vi "概率随机数生成.vi"(10 "数值比例":string, 11 "数值范围":string) -> (0 "浮点数（字符串）":string, 1 "整数（字符串）":string, 2 "浮点数":dbl, 3 "整数":i32)   [LabVIEW 2013]
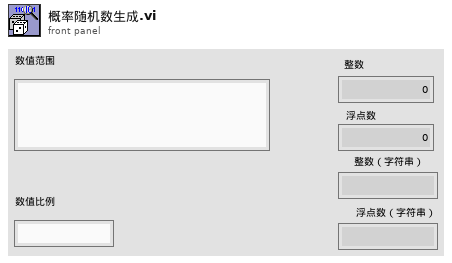
[diagram p1: front panel]
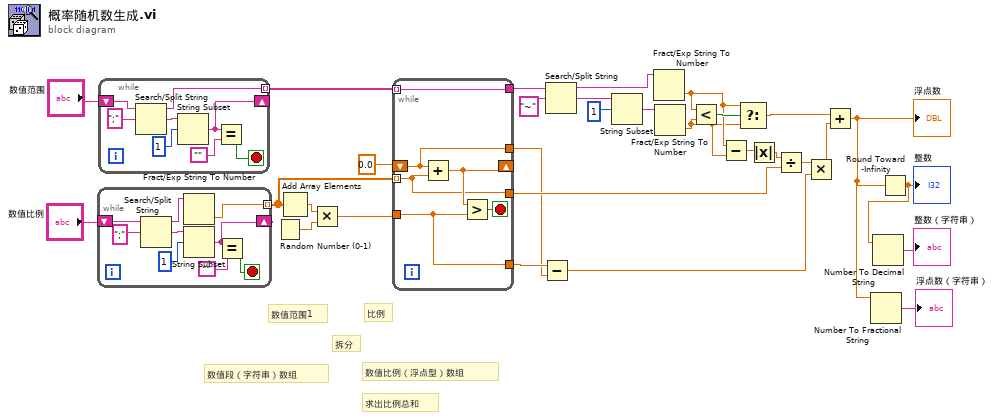
[diagram p0: block diagram]
diagram:
  # "求出比例总和"
  # "数值比例（浮点型）数组"
  # "数值段（字符串）数组"
  # "拆分"
  # "比例"
  # "数值范围1"
  n1 = while {
    tunnel: [w36] -> w26 mode=indexing
    shift-right: [w33] -> _
    shift-left: "数值比例" -> [w39]
    stop <- w31 stop-if-true
    n2 = Search/Split String(string=w39, search string/char (-)=";" ("搜索字符串/字符(-)")) -> (substring before match=w37:string, match + rest of string=w35:string)  [unwired: 1 in, 1 out]
    n3 = Fract/Exp String To Number(string=w37) -> (number=w36:dbl)  [unwired: 3 in, 1 out]
    n4 = String Subset(string=w35, offset (0)=1 ("偏移量(0)")) -> (substring=w33:string)  [unwired: 1 in]
    n5 = Equal?(x=w33, y="") -> (x = y?=w31:bool)
  }
  n6 = while {
    shift-right: [w43] -> _
    shift-left: "数值范围" -> [w47]
    tunnel: [w40] -> w23 mode=indexing
    stop <- w41 stop-if-true
    n7 = Search/Split String(string=w47, search string/char (-)=";" ("搜索字符串/字符(-)")) -> (substring before match=w40:string, match + rest of string=w45:string)  [unwired: 1 in, 1 out]
    n8 = String Subset(string=w45, offset (0)=1 ("偏移量(0)")) -> (substring=w43:string)  [unwired: 1 in]
    n9 = Equal?(x=w43, y="") -> (x = y?=w41:bool)
  }
  n10 = Random Number (0-1)() -> (number: 0 to 1=w27:dbl)
  n11 = Add Array Elements(numeric array=w26) -> (sum=w28:dbl)
  n12 = Multiply(x=w28, y=w27) -> (x*y=w24:dbl)
  n13 = while {
    tunnel: w24 -> [w50]
    tunnel: w26 -> [w49] mode=indexing
    shift-right: [w52] -> _
    shift-left: 0.0 -> [w48]
    tunnel: w23 -> [w51] mode=indexing
    tunnel: [w51] -> w22
    tunnel: [w50] -> w7
    tunnel: [w49] -> w10
    tunnel: [w48] -> w6
    stop <- w53 stop-if-true
    n14 = Add(x=w48, y=w49) -> (x+y=w52:dbl)
    n15 = Greater?(x=w52, y=w50) -> (0:w53:bool)
  }
  n16 = Subtract(x=w7, y=w6) -> (x-y=w5:dbl)
  n17 = Search/Split String(string=w22, search string/char (-)="~" ("搜索字符串/字符(-)")) -> (substring before match=w16:string, match + rest of string=w20:string)  [unwired: 1 in, 1 out]
  n18 = String Subset(string=w20, offset (0)=1 ("偏移量(0)")) -> (substring=w18:string)  [unwired: 1 in]
  n19 = Fract/Exp String To Number(string=w16) -> (number=w14:dbl)  [unwired: 3 in, 1 out]
  n20 = Fract/Exp String To Number(string=w18) -> (number=w13:dbl)  [unwired: 3 in, 1 out]
  n21 = Less?(x=w14, y=w13) -> (x < y?=w17:bool)
  n22 = Subtract(x=w14, y=w13) -> (x-y=w12:dbl)
  n23 = Select(t=w14, s=w17, f=w13) -> (s? t:f=w15:dbl)
  n24 = Absolute Value(x=w12) -> (abs(x)=w11:dbl)
  n25 = Divide(x=w11, y=w10) -> (x/y=w9:dbl)
  n26 = Multiply(x=w9, y=w5) -> (x*y=w8:dbl)
  n27 = Add(x=w15, y=w8) -> (x+y=w1:dbl)
  "浮点数" <- w1
  n28 = Number To Fractional String(number=w1) -> (F-format string=→"浮点数（字符串）":string)  [unwired: 3 in]
  n29 = Round Toward -Infinity(1:w1) -> (0:w4:dbl)
  "整数" <- w4
  n30 = Number To Decimal String(number=w4) -> (decimal integer string=→"整数（字符串）":string)  [unwired: 1 in]
